vi "alpha-0.1.0.vi"() -> ()   [LabVIEW 2016]
uses:
  <vilib>/FPGAPlugInAG/cRIO-9063/niLvFpga_Open_cRIO-9063.vi
  <vilib>/rvi/interface/common/dynamic/niFpgaDynamicAddResources.vi
  <vilib>/Utility/error.llb/Error Cluster From Error Code.vi
  <vilib>/rvi/errors/niLvFpgaAdjustHostInterfaceError.vi
  <vilib>/FPGAPlugInAG/Dynamic/niLvFpga_Close_Dynamic.vi
  <vilib>/rvi/interface/nirviOpenFPGA/nirviOpenFPGA.xnode
  FPGA Bitfiles/multi-functionpr_FPGATarget_DI&AO_PaHU11gpxn0.lvbitx
  DI&AO.vi
  <vilib>/rvi/interface/nirviReadWriteControl/nirviReadWriteControl.xnode
  <vilib>/rvi/interface/nirviCloseFPGA/nirviCloseFPGA.xnode
  NiFpgaLv.dll
  <vilib>/rvi/interface/Simulation/niFpgaSimulationCallBeginRW.vi
panel:
  out "Mod2/DIO3":bool
  out "Mod2/DIO2":bool
  in  "end1":dbl=5.0 format="%#_13g"
  in  "begin1":dbl format="%#_13g"
  in  "step1":dbl=1.0 format="%#_13g"
  in  "OUT1":T1(ring)
  in  "step":dbl=1.0 format="%#_13g"
  in  "begin":dbl format="%#_13g"
  in  "end":dbl=5.0 format="%#_13g"
  out "IN0 & IN1":bool[](array[boolean])
  in  "OUT0":T1(ring)
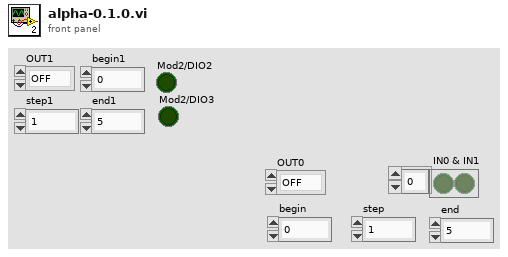
[diagram p1: front panel]
types:
  T1 = enum16{"OFF", "SWITCH", "AND GATE", "OR GATE", "ITERATION"}
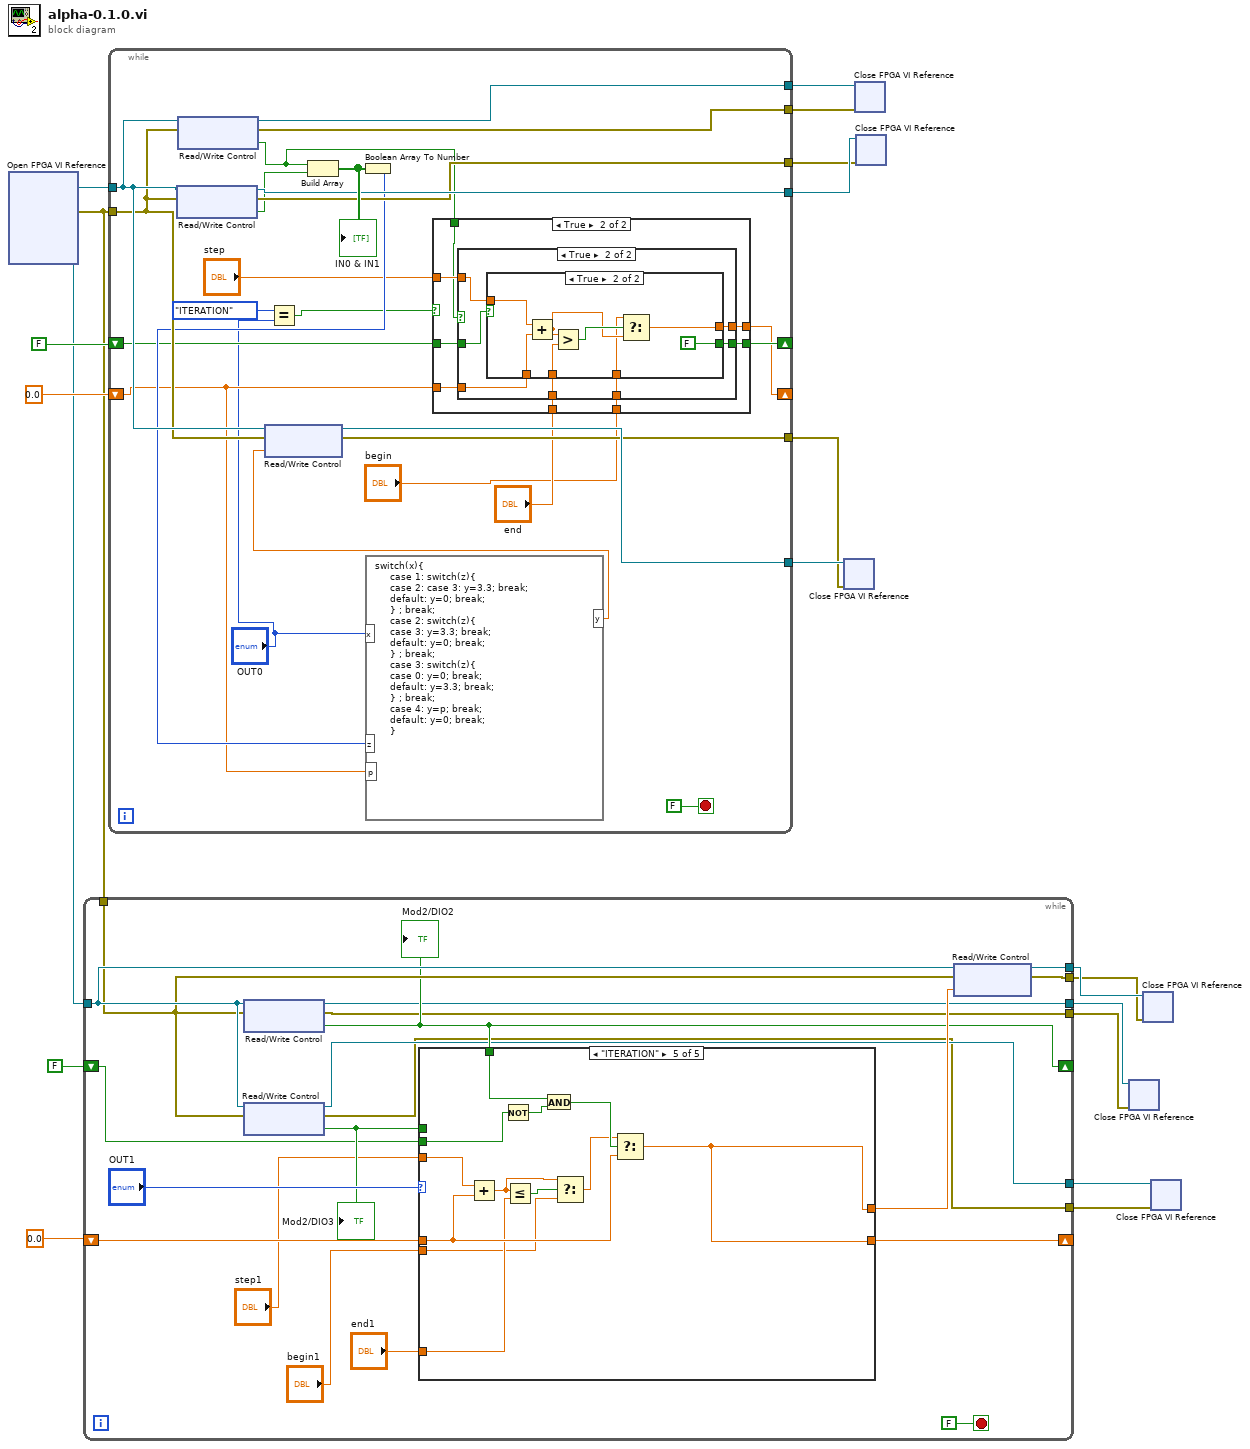
[diagram p0: block diagram]
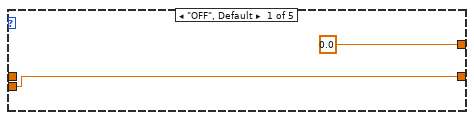
[diagram p2: hidden frame]
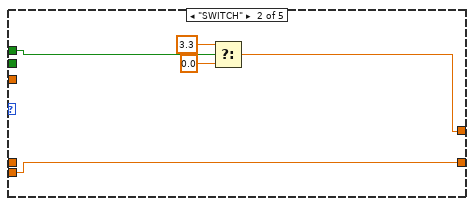
[diagram p3: hidden frame]
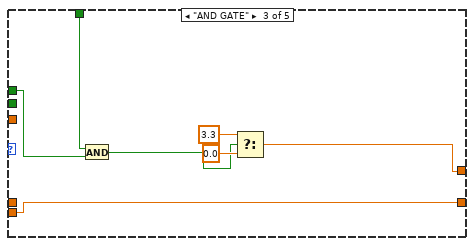
[diagram p4: hidden frame]
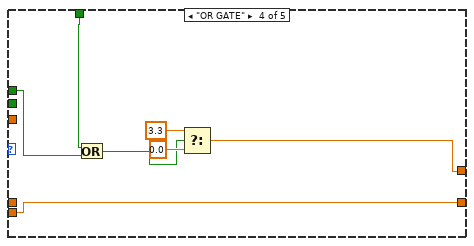
[diagram p5: hidden frame]
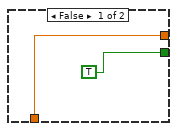
[diagram p6: hidden frame]
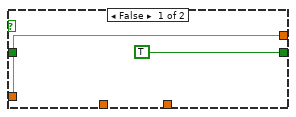
[diagram p7: hidden frame]
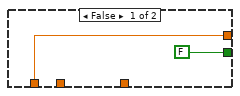
[diagram p8: hidden frame]
diagram:
  n1 = xnode "Open FPGA VI Reference"() -> ("FPGA VI Reference Out"=w10:refnum<k20>, "error out"=w9:errorcluster)  [unwired: 2 in]
  n2 = while {
    tunnel: w10 -> [w35]
    tunnel: w9 -> [w34]
    shift-right: [w27] -> _
    shift-left: 0.0 -> [w29]
    shift-right: [w31] -> _
    shift-left: FALSE -> [w30]
    tunnel: [w24] -> w6
    tunnel: [w23] -> w5
    tunnel: [w22] -> w4
    tunnel: [w21] -> w3
    tunnel: [w20] -> w2
    tunnel: [w19] -> w1
    stop <- FALSE stop-if-true
    n3 = xnode "Read/Write Control"("FPGA VI Reference In"=w35, "error in"=w34) -> ("FPGA VI Reference Out"=w22:refnum<k20>, "error out"=w21:errorcluster, "Mod2/DIO2"=w31:bool)
    "Mod2/DIO2" <- w31
    n4 = xnode "Read/Write Control"("FPGA VI Reference In"=w35, "error in"=w34) -> ("FPGA VI Reference Out"=w24:refnum<k20>, "error out"=w23:errorcluster, "Mod2/DIO3"=w33:bool)
    "Mod2/DIO3" <- w33
    n5 = case shown="\"ITERATION\"" "OUT1" {
      tunnel: w33 -> [_ w44 w50 w57 _]
      tunnel: [0.0 w41 w46 w53 w65] -> w32
      tunnel: w31 -> [_ _ w51 w58 w68]
      tunnel: w30 -> [_ _ _ _ w70]
      tunnel: w29 -> [_ _ _ _ w64]
      tunnel: "step1" -> [_ _ _ _ w66]
      tunnel: [w38 w40 w45 w52 w65] -> w27
      tunnel: "begin1" -> [w38 w40 w45 w52 w60]
      tunnel: "end1" -> [_ _ _ _ w63]
      frame "OFF", Default {
      }
      frame "SWITCH" {
        n6 = Select(t=3.3, s=w44, f=0.0) -> (s? t:f=w41:dbl)
      }
      frame "AND GATE" {
        n7 = And(x=w51, y=w50) -> (x .and. y?=w47:bool)
        n8 = Select(t=3.3, s=w47, f=0.0) -> (s? t:f=w46:dbl)
      }
      frame "OR GATE" {
        n9 = Or(x=w58, y=w57) -> (x .or. y?=w54:bool)
        n10 = Select(t=3.3, s=w54, f=0.0) -> (s? t:f=w53:dbl)
      }
      frame "ITERATION" {
        n11 = Add(x=w66, y=w64) -> (x+y=w61:dbl)
        n12 = Not(x=w70) -> (.not. x?=w69:bool)
        n13 = Less Or Equal?(x=w61, y=w63) -> (x <= y?=w62:bool)
        n14 = And(x=w68, y=w69) -> (x .and. y?=w67:bool)
        n15 = Select(t=w61, s=w62, f=w60) -> (s? t:f=w59:dbl)
        n16 = Select(t=w59, s=w67, f=w64) -> (s? t:f=w65:dbl)
      }
    }
    n17 = xnode "Read/Write Control"("FPGA VI Reference In"=w35, "error in"=w34, "Mod4/AO1"=w32) -> ("FPGA VI Reference Out"=w20:refnum<k20>, "error out"=w19:errorcluster)
  }
  n18 = while {
    tunnel: w10 -> [w85]
    tunnel: w9 -> [w84]
    tunnel: [w91] -> w18
    tunnel: [w90] -> w17
    tunnel: [w89] -> w16
    tunnel: [w88] -> w15
    tunnel: [w87] -> w14
    tunnel: [w86] -> w13
    shift-right: [w80] -> _
    shift-left: FALSE -> [w81]
    shift-right: [w77] -> _
    shift-left: 0.0 -> [w76]
    stop <- FALSE stop-if-true
    n19 = xnode "Read/Write Control"("FPGA VI Reference In"=w85, "error in"=w84) -> ("FPGA VI Reference Out"=w89:refnum<k20>, "error out"=w88:errorcluster, "Mod2/DIO1"=w83:bool)
    n20 = xnode "Read/Write Control"("FPGA VI Reference In"=w85, "error in"=w84) -> ("FPGA VI Reference Out"=w91:refnum<k20>, "error out"=w90:errorcluster, "Mod2/DIO0"=w72:bool)
    n21 = Equal?(x=T1."ITERATION", y="OUT0") -> (x = y?=w73:bool)
    n22 = Build Array(w72, w83) -> (w92:bool[])
    "IN0 & IN1" <- w92
    n23 = Boolean Array To Number(Boolean array=w92) -> (number=w82:u32)
    n24 = formula code="switch(x){ \n     case 1: switch(z){ \n     case 2: case 3: y=3.3; break; \n     default: y=0; break; \n     } ; break; \n     case 2: switch(z){ \n     case 3: y=3.3; break; \n     default: y=0; break; \n     } ; break;\n     case 3: switch(z){ \n     case 0: y=0; break; \n     default: y=3.3; break; \n     } ; break;\n     case 4: y=p; break;  \n     default: y=0; break; \n     }"("x"="OUT0", "z"=w82, "p"=w76) -> ("y"=w93:dbl)
    n25 = xnode "Read/Write Control"("FPGA VI Reference In"=w85, "error in"=w84, "Mod4/AO0"=w93) -> ("FPGA VI Reference Out"=w87:refnum<k20>, "error out"=w86:errorcluster)
    n26 = case shown="True" w73 {
      tunnel: w81 -> [_ w104]
      tunnel: [TRUE w103] -> w80
      tunnel: "step" -> [_ w102]
      tunnel: "end" -> [_ w101]
      tunnel: [w95 w100] -> w77
      tunnel: "begin" -> [w95 w99]
      tunnel: w76 -> [_ w98]
      tunnel: w72 -> [_ w97]
      frame False {
      }
      frame True {
        n27 = case shown="True" w97 {
          tunnel: w104 -> [_ w113]
          tunnel: [TRUE w112] -> w103
          tunnel: w102 -> [_ w111]
          tunnel: w98 -> [w105 w110]
          tunnel: w101 -> [_ w109]
          tunnel: [w105 w108] -> w100
          tunnel: w99 -> [_ w107]
          frame False {
          }
          frame True {
            n28 = case shown="True" w113 {
              tunnel: [FALSE FALSE] -> w112
              tunnel: w111 -> [_ w122]
              tunnel: w110 -> [w114 w119]
              tunnel: w109 -> [_ w121]
              tunnel: [w114 w117] -> w108
              tunnel: w107 -> [_ w116]
              frame False {
              }
              frame True {
                n29 = Add(x=w122, y=w119) -> (x+y=w118:dbl)
                n30 = Greater?(x=w118, y=w121) -> (0:w120:bool)
                n31 = Select(t=w116, s=w120, f=w118) -> (s? t:f=w117:dbl)
              }
            }
          }
        }
      }
    }
  }
  n32 = xnode "Close FPGA VI Reference"("FPGA VI Reference In"=w14, "error in"=w13) -> ()  [unwired: 1 out]
  n33 = xnode "Close FPGA VI Reference"("FPGA VI Reference In"=w18, "error in"=w17) -> ()  [unwired: 1 out]
  n34 = xnode "Close FPGA VI Reference"("FPGA VI Reference In"=w16, "error in"=w15) -> ()  [unwired: 1 out]
  n35 = xnode "Close FPGA VI Reference"("FPGA VI Reference In"=w4, "error in"=w3) -> ()  [unwired: 1 out]
  n36 = xnode "Close FPGA VI Reference"("FPGA VI Reference In"=w2, "error in"=w1) -> ()  [unwired: 1 out]
  n37 = xnode "Close FPGA VI Reference"("FPGA VI Reference In"=w6, "error in"=w5) -> ()  [unwired: 1 out]
